vi "GetSensorStatue.vi"() -> ()   [LabVIEW 2011]
uses:
  API/API DYM.lvlib
panel:
  out "array output":i32[](array[numeric])
  in  "获取传感器状态按钮":bool
  out "布尔":bool
  in  "启动按钮":bool
  in  "退出按钮":bool
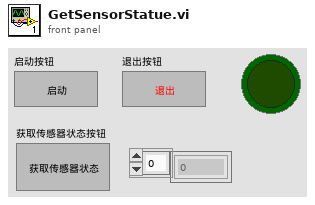
[diagram p1: front panel]
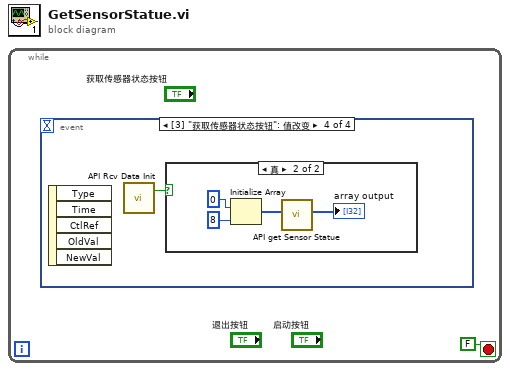
[diagram p0: block diagram]
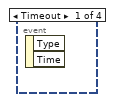
[diagram p2: hidden frame]
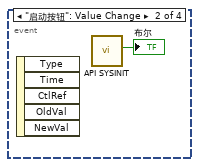
[diagram p3: hidden frame]
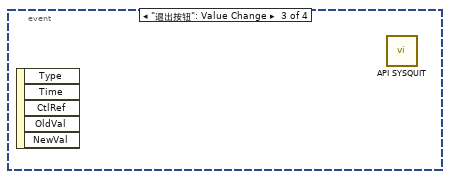
[diagram p4: hidden frame]
diagram:
  n1 = while {
    stop <- FALSE stop-if-true
    n2 = event shown="[3] \"获取传感器状态按钮\": 值改变" {
      selector: _ -> [_ _ _ _]
      dyn-events: _ -> [_ _ _ _]
      timeout: _ -> [_ _ _ _]
      event Timeout {
        n3 = event-data() -> ()  [unwired: 1 in, 2 out]
      }
      event "启动按钮": Value Change {
        n4 = event-data() -> ()  [unwired: 1 in, 5 out]
        n5 = call "API SYSINIT.vi"() -> ("SYSINIT return value"=→"布尔":bool)  [unwired: 11 in]
      }
      event "退出按钮": Value Change {
        n6 = event-data() -> ()  [unwired: 1 in, 5 out]
        n7 = call "API SYSQUIT.vi"() -> ()  [unwired: 12 in]
      }
      event "获取传感器状态按钮": Value Change {
        n8 = event-data() -> ()  [unwired: 1 in, 5 out]
        n9 = call "API Rcv Data Init.vi"() -> ("RTV"=w3:bool)  [unwired: 2 in, 1 out]
        n10 = case shown="真" w3 {
          frame False {
          }
          frame True {
            n11 = Initialize Array(0 ("元素"), 8 ("维数大小")) -> (w5:i32[])
            n12 = call "API get Sensor Statue.vi"("array input"=w5) -> ("array output"=→"array output":i32[])  [unwired: 9 in, 1 out]
          }
        }
      }
    }
  }
